vi "Setup Statically-Linked subWorkers.vi"(8 "error in":errorcluster, 11 "TopUI in":refnum<class "TopUI.lvclass">) -> (0 "error out":errorcluster, 3 "TopUI out":refnum<class "TopUI.lvclass">)   [LabVIEW 2025, in "TopUI.lvclass"]
doc: "This VI performs a setup of all the statically-linked subWorkers that belong to the Worker that owns this VI. This VI must be called <b>before</b> any statically-linked subWorkers are called."
uses:
  TopUI.lvclass
  TopUI.lvclass/TopUI.ctl
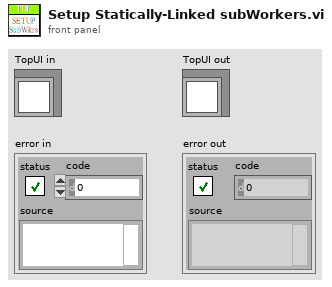
[diagram p1: front panel]
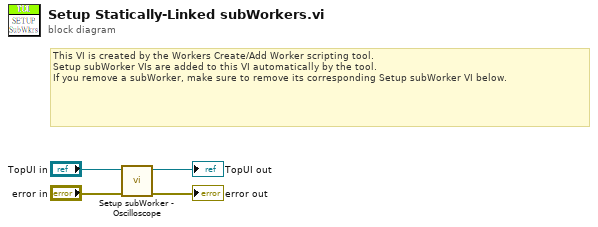
[diagram p0: block diagram]
diagram:
  # "This VI is created by the Workers Create/Add Worker scripting tool.\nSetup subWorker VIs are added to this VI automatically by the tool.\nIf you remove a subWorker, make sure to remove its corresponding Setup subWorker VI below."
  n1 = call "Setup subWorker - Oscilloscope.vi"("error in"="error in", "TopUI in"="TopUI in") -> ("error out"=→"error out":errorcluster, "TopUI out"=→"TopUI out":refnum<class "TopUI.lvclass">)  [unwired: 8 in]
